vi "test_dragon_file--get_version_in_subtable.vi"(8 "error in (no error)":errorcluster) -> (0 "error out":errorcluster)   [LabVIEW 2020]
uses:
  toml/toml.lvclass
  <vilib>/addons/_JKI Toolkits/Caraya/classes/Assert/Assert.lvclass
  <vilib>/addons/_JKI Toolkits/Caraya/classes/Test/Test.lvclass
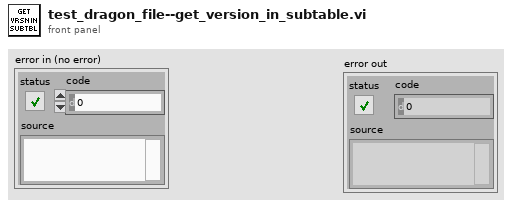
[diagram p1: front panel]
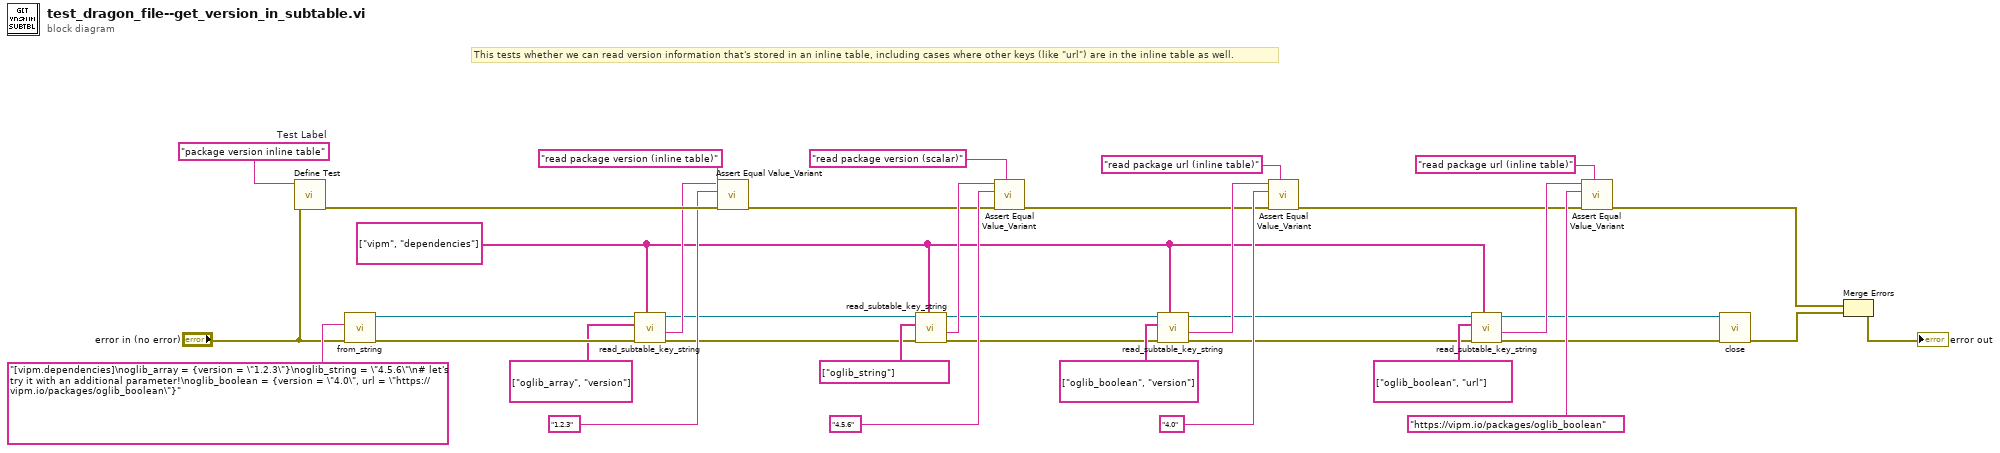
[diagram p0: block diagram]
diagram:
  w2 = string[] ["vipm", "dependencies"]
  w33 = "package version inline table"  # Test Label
  # "This tests whether we can read version information that's stored in an inline table, including cases where other keys (like \"url\") are in the inline table as well."
  n1 = call <vilib>:"Define Test.vi"("error in (no error)"="error in (no error)", "Label (VI Title)"=w33) -> ("error out"=w34:errorcluster)  [unwired: 9 in]
  n2 = call "from_string.vi"("error in (no error)"="error in (no error)", "toml"="[vipm.dependencies]\noglib_array = {version = \"1.2.3\"}\noglib_string = \"4.5.6\"\n# let's try it with an additional parameter!\noglib_boolean = {version = \"4.0\", url = \"https://vipm.io/packages/oglib_boolean\"}" ("toml_string in")) -> ("error out"=w31:errorcluster, "toml out"=w32:refnum<class "toml.lvclass">)  [unwired: 8 in]
  n3 = call "read_subtable_key_string.vi"("subtables"=w2, "error in (no error)"=w31, "subkeys"=string[] ["oglib_array", "version"], "toml in"=w32) -> ("error out"=w19:errorcluster, "value"=w28:string, "toml out"=w20:refnum<class "toml.lvclass">)  [unwired: 4 in, 1 out]
  n4 = call <vilib>:"Assert Equal Value_Variant.vi"("Label"="read package version (inline table)", "error in (no error)"=w34, "Y"="1.2.3" ("table_name"), "X"=w28) -> ("error out"=w21:errorcluster)  [unwired: 7 in]
  n5 = call "read_subtable_key_string.vi"("subtables"=w2, "error in (no error)"=w19, "subkeys"=string[] ["oglib_string"], "toml in"=w20) -> ("error out"=w6:errorcluster, "value"=w23:string, "toml out"=w5:refnum<class "toml.lvclass">)  [unwired: 4 in, 1 out]
  n6 = call <vilib>:"Assert Equal Value_Variant.vi"("Label"="read package version (scalar)", "error in (no error)"=w21, "Y"="4.5.6" ("table_name"), "X"=w23) -> ("error out"=w7:errorcluster)  [unwired: 7 in]
  n7 = call "read_subtable_key_string.vi"("subtables"=w2, "error in (no error)"=w6, "subkeys"=string[] ["oglib_boolean", "version"], "toml in"=w5) -> ("error out"=w3:errorcluster, "value"=w9:string, "toml out"=w4:refnum<class "toml.lvclass">)  [unwired: 4 in, 1 out]
  n8 = call <vilib>:"Assert Equal Value_Variant.vi"("Label"="read package url (inline table)", "error in (no error)"=w7, "Y"="4.0" ("table_name"), "X"=w9) -> ("error out"=w1:errorcluster)  [unwired: 7 in]
  n9 = call "read_subtable_key_string.vi"("subtables"=w2, "error in (no error)"=w3, "subkeys"=string[] ["oglib_boolean", "url"], "toml in"=w4) -> ("error out"=w13:errorcluster, "value"=w17:string, "toml out"=w12:refnum<class "toml.lvclass">)  [unwired: 4 in, 1 out]
  n10 = call <vilib>:"Assert Equal Value_Variant.vi"("Label"="read package url (inline table)", "error in (no error)"=w1, "Y"="https://vipm.io/packages/oglib_boolean" ("table_name"), "X"=w17) -> ("error out"=w14:errorcluster)  [unwired: 7 in]
  n11 = call "close.vi"("error in (no error)"=w13, "toml in"=w12) -> ("error out"=w30:errorcluster)  [unwired: 9 in]
  n12 = Merge Errors(w14, w30) -> (→"error out":errorcluster)
